vi "Register gRPC Methods.vi"(8 "error in (no error)":errorcluster, 11 "Template Server in":refnum<class "TestServer.lvclass">) -> (0 "error out":errorcluster, 3 "Template Server out":refnum<class "TestServer.lvclass">)   [LabVIEW 2019, in "TestServer.lvlib" / "TestServer.lvclass"]
uses:
  TestServer.lvclass
  typeDefs/Server Internal UEs.ctl
  typeDefs/Server Internal Message.ctl
  typeDefs/Server gRPC UEs.ctl
  gRPC lvSupport/Server API/typeDefs/gRPCId Cluster.ctl
  gRPC lvSupport/Server API/typeDefs/grpcId.ctl
  TestServer.lvclass/TestServer.ctl
  gRPC lvSupport/gprc-lvsupport.lvlib
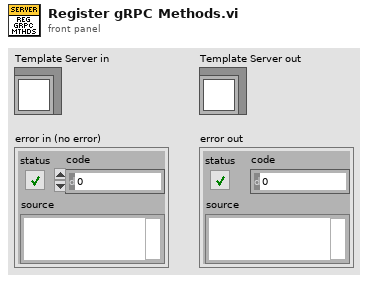
[diagram p1: front panel]
types:
  T1 = typedef "TestServer.lvlib/TestServer.lvclass/Server gRPC UEs.ctl" = cluster{"StreamLatencyTest gRPC UE":refnum<user-event>, "StreamLatencyTestClient gRPC UE":refnum<user-event>, "StreamLatencyTestServer gRPC UE":refnum<user-event>, "Init gRPC UE":refnum<user-event>, "InitWithOptions gRPC UE":refnum<user-event>, "AutoSetup gRPC UE":refnum<user-event>, "ConfigureHorizontalTiming gRPC UE":refnum<user-event>, "TestWrite gRPC UE":refnum<user-event>, "Read gRPC UE":refnum<user-event>, "ReadContinuously gRPC UE":refnum<user-event>}
  T2 = typedef "TestServer.lvlib/TestServer.lvclass/Server Internal UEs.ctl" = cluster{"StreamLatencyTest Internal UE":refnum<user-event>, "StreamLatencyTestClient Internal UE":refnum<user-event>, "StreamLatencyTestServer Internal UE":refnum<user-event>, "Init Internal UE":refnum<user-event>, "InitWithOptions Internal UE":refnum<user-event>, "AutoSetup Internal UE":refnum<user-event>, "ConfigureHorizontalTiming Internal UE":refnum<user-event>, "TestWrite Internal UE":refnum<user-event>, "Read Internal UE":refnum<user-event>, "ReadContinuously Internal UE":refnum<user-event>}
  T3 = typedef "TestServer.lvlib/gprc-lvsupport.lvlib/grpcId.ctl" = u64
  T4 = typedef "TestServer.lvlib/TestServer.lvclass/Server Internal Message UE.ctl" = refnum<user-event>
  T5 = typedef "TestServer.lvlib/gprc-lvsupport.lvlib/gRPCId Cluster UE.ctl" = refnum<user-event>
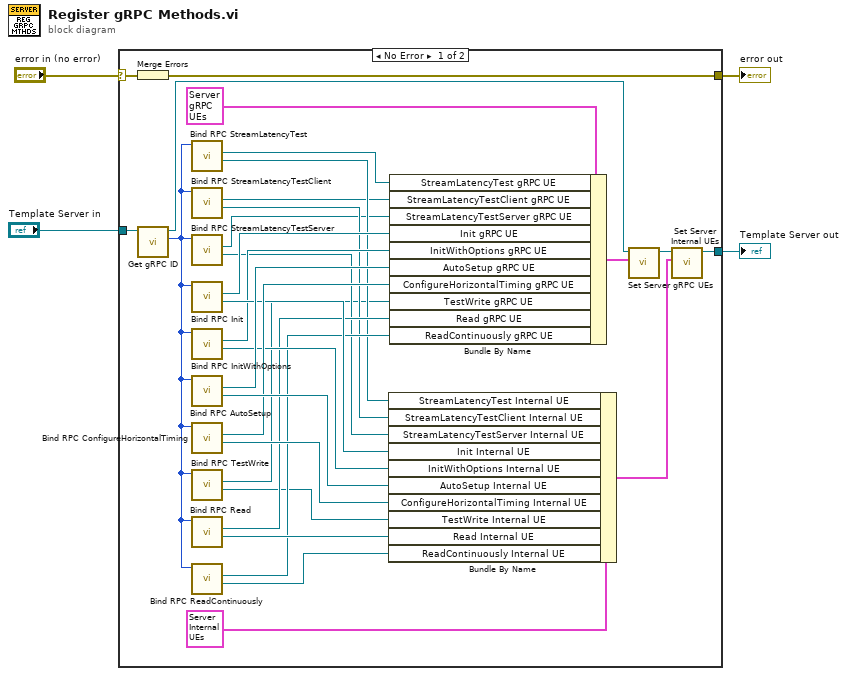
[diagram p0: block diagram]
diagram:
  n1 = case shown="No Error" "error in (no error)" {
    selector: "error in (no error)" -> [w26 w36]
    tunnel: "Template Server in" -> [w34 w37]
    tunnel: [w33 w36] -> w3
    tunnel: [w32 w37] -> w2
    frame No Error {
      n2 = Merge Errors(w26) -> (w33:errorcluster)
      n3 = call "Get gRPC ID.vi"("OOP Server in"=w34) -> ("gRPC ID"=w25:T3, "OOP Server out"=w35:refnum<class "TestServer.lvclass">)  [unwired: 9 in]
      n4 = call "Bind RPC StreamLatencyTest.vi"("gRPCid server in"=w25) -> ("StreamLatencyTest Internal UE"=w12:T4, "StreamLatencyTest gRPC UE"=w11:T5)  [unwired: 7 in, 2 out]
      n5 = call "Bind RPC StreamLatencyTestClient.vi"("gRPCid server in"=w25) -> ("StreamLatencyTestClient Internal UE"=w10:T4, "StreamLatencyTestClient gRPC UE"=w9:T5)  [unwired: 7 in, 2 out]
      n6 = call "Bind RPC StreamLatencyTestServer.vi"("gRPCid server in"=w25) -> ("StreamLatencyTestServer Internal UE"=w8:T4, "StreamLatencyTestServer gRPC UE"=w7:T5)  [unwired: 7 in, 2 out]
      n7 = call "Bind RPC Init.vi"("gRPCid server in"=w25) -> ("Init Internal UE"=w20:T4, "Init gRPC UE"=w19:T5)  [unwired: 7 in, 2 out]
      n8 = call "Bind RPC InitWithOptions.vi"("gRPCid server in"=w25) -> ("InitWithOptions Internal UE"=w18:T4, "InitWithOptions gRPC UE"=w17:T5)  [unwired: 7 in, 2 out]
      n9 = call "Bind RPC AutoSetup.vi"("gRPCid server in"=w25) -> ("AutoSetup Internal UE"=w24:T4, "AutoSetup gRPC UE"=w23:T5)  [unwired: 7 in, 2 out]
      n10 = call "Bind RPC ConfigureHorizontalTiming.vi"("gRPCid server in"=w25) -> ("ConfigureHorizontalTiming Internal UE"=w22:T4, "ConfigureHorizontalTiming gRPC UE"=w21:T5)  [unwired: 7 in, 2 out]
      n11 = call "Bind RPC TestWrite.vi"("gRPCid server in"=w25) -> ("TestWrite Internal UE"=w6:T4, "TestWrite gRPC UE"=w5:T5)  [unwired: 7 in, 2 out]
      n12 = call "Bind RPC Read.vi"("gRPCid server in"=w25) -> ("Read Internal UE"=w16:T4, "Read gRPC UE"=w15:T5)  [unwired: 7 in, 2 out]
      n13 = call "Bind RPC ReadContinuously.vi"("gRPCid server in"=w25) -> ("ReadContinuously Internal UE"=w14:T4, "ReadContinuously gRPC UE"=w13:T5)  [unwired: 7 in, 2 out]
      n14 = Bundle By Name ("Bundle Internal UEs")(cluster=T2 {"StreamLatencyTest Internal UE"=refnum, "StreamLatencyTestClient Internal UE"=refnum, "StreamLatencyTestServer Internal UE"=refnum, "Init Internal UE"=refnum, "InitWithOptions Internal UE"=refnum, "AutoSetup Internal UE"=refnum, "ConfigureHorizontalTiming Internal UE"=refnum, "TestWrite Internal UE"=refnum, "Read Internal UE"=refnum, "ReadContinuously Internal UE"=refnum} ("Server Internal UEs"), "StreamLatencyTest Internal UE"=w12, "StreamLatencyTestClient Internal UE"=w10, "StreamLatencyTestServer Internal UE"=w8, "Init Internal UE"=w20, "InitWithOptions Internal UE"=w18, "AutoSetup Internal UE"=w24, "ConfigureHorizontalTiming Internal UE"=w22, "TestWrite Internal UE"=w6, "Read Internal UE"=w16, "ReadContinuously Internal UE"=w14) -> (w31:T2)
      n15 = Bundle By Name ("Bundle gRPC UEs")(cluster=T1 {"StreamLatencyTest gRPC UE"=refnum, "StreamLatencyTestClient gRPC UE"=refnum, "StreamLatencyTestServer gRPC UE"=refnum, "Init gRPC UE"=refnum, "InitWithOptions gRPC UE"=refnum, "AutoSetup gRPC UE"=refnum, "ConfigureHorizontalTiming gRPC UE"=refnum, "TestWrite gRPC UE"=refnum, "Read gRPC UE"=refnum, "ReadContinuously gRPC UE"=refnum} ("gRPC Server Method Events"), "StreamLatencyTest gRPC UE"=w11, "StreamLatencyTestClient gRPC UE"=w9, "StreamLatencyTestServer gRPC UE"=w7, "Init gRPC UE"=w19, "InitWithOptions gRPC UE"=w17, "AutoSetup gRPC UE"=w23, "ConfigureHorizontalTiming gRPC UE"=w21, "TestWrite gRPC UE"=w5, "Read gRPC UE"=w15, "ReadContinuously gRPC UE"=w13) -> (w28:T1)
      n16 = call "Set Server gRPC UEs.vi"("Server gRPC UEs"=w28, "OOP Server in"=w35) -> ("OOP Server out"=w29:refnum<class "TestServer.lvclass">)  [unwired: 9 in]
      n17 = call "Set Server Internal UEs.vi"("Server Internal UEs"=w31, "OOP Server in"=w29) -> ("OOP Server out"=w32:refnum<class "TestServer.lvclass">)  [unwired: 9 in]
    }
    frame Error {
    }
  }
  "error out" <- w3
  "Template Server out" <- w2
